vi "Swap_Boolean[].vi"(4 "Swap(T)":bool=TRUE, 6 "b":bool[](array[boolean]), 7 "a":bool[](array[boolean])) -> (1 "b":bool[](array[boolean]), 2 "a":bool[](array[boolean]))   [LabVIEW 2012]
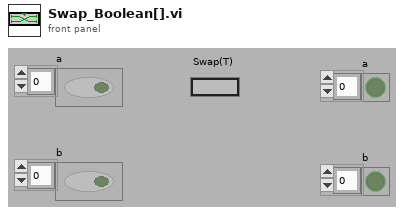
[diagram p1: front panel]
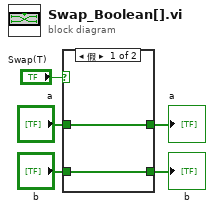
[diagram p0: block diagram]
diagram:
  n1 = case shown="假" "Swap(T)" {
    tunnel: "a" -> [w7 w9]
    tunnel: "b" -> [w6 w8]
    tunnel: [w7 w8] -> w2
    tunnel: [w6 w9] -> w1
    frame False {
    }
    frame True {
    }
  }
  "a" <- w2
  "b" <- w1
